vi "test appel.vi"() -> ()   [LabVIEW 2011]
uses:
  My DLL/Ap_int_usb.dll
panel:
  in  "Stop Button":bool
  out "Graphe":u16[](graph)
  out "Version DLL":i32
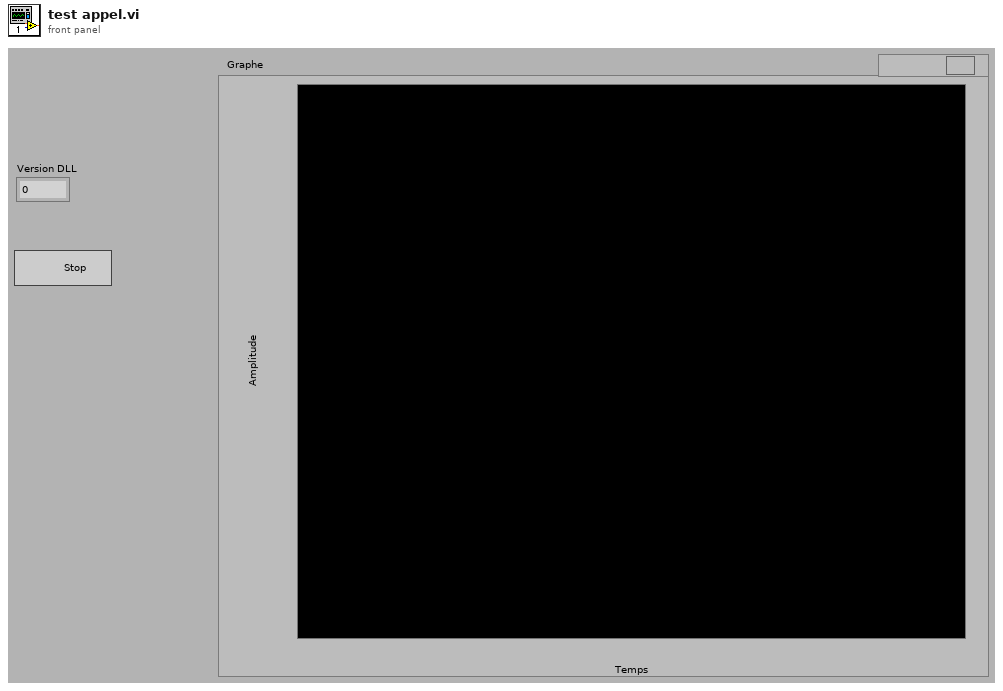
[diagram p1: front panel]
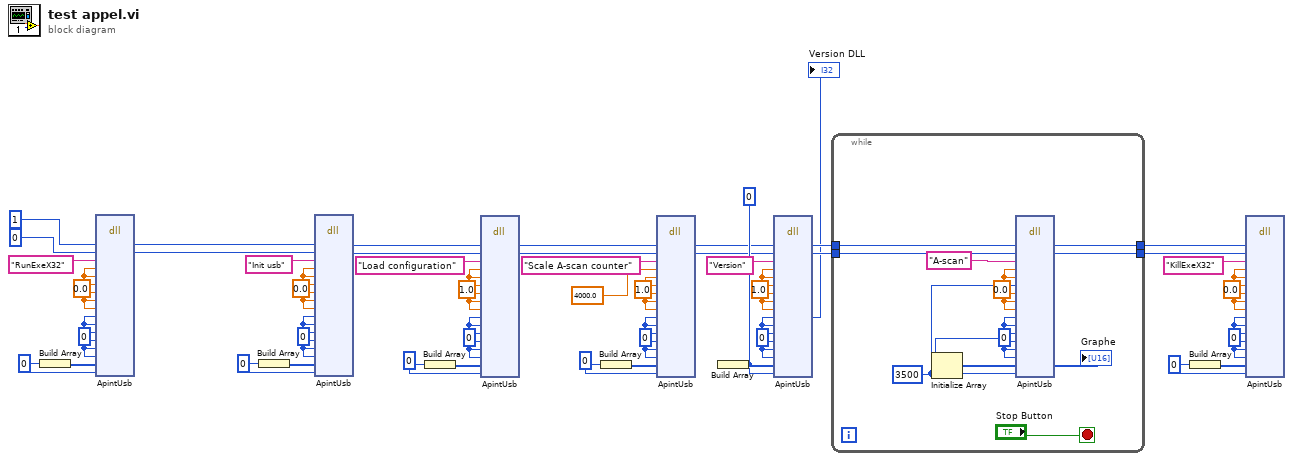
[diagram p0: block diagram]
diagram:
  w7 = u16 0 ("élément")
  w9 = i16 0 ("Out1")
  w10 = 1.0 ("In1")
  w14 = u16 0 ("élément")
  w16 = i16 0 ("Out1")
  w17 = 0.0 ("In1")
  w22 = u16 0 ("élément")
  w24 = i16 0 ("Out1")
  w25 = 0.0 ("In1")
  w30 = u16 0 ("élément")
  w32 = i16 0 ("Out1")
  w33 = 1.0 ("In1")
  w35 = u16 0 ("élément")
  w39 = i16 0 ("Out1")
  w40 = 1.0 ("In1")
  w42 = u16 0 ("élément")
  w44 = i16 0 ("Out1")
  w45 = 0.0 ("In1")
  n1 = Build Array(w22) -> (w23:u16[])
  n2 = dll-call lib="C:/Labview/Madelin/V2     LV2011 x64/DLL_Ap_int_usb   LV2011 x64/My DLL/Ap_int_usb.dll" fn="ApintUsb"("ProductNumber"=u32 1, "ChannelNumber"=u32 0, "Function"="RunExeX32", "In1"=w25, "In2"=w25, "In3"=w25, "In4"=w25, "In5"=w25, "In6"=w25, "Out1"=w24, "Out2"=w24, "Out3"=w24, "Out4"=w24, "Out5"=w24, "Out6"=w24, "Array"=w23, "Len"=w22) -> ("ProductNumber"=w19:u32, "ChannelNumber"=w1:u32)  [unwired: 19 in, 2 out]
  n3 = Build Array(w42) -> (w43:u16[])
  n4 = dll-call lib="C:/Labview/Madelin/V2     LV2011 x64/DLL_Ap_int_usb   LV2011 x64/My DLL/ap_int_usb.dll" fn="ApintUsb"("ProductNumber"=w19, "ChannelNumber"=w1, "Function"="Init usb", "In1"=w45, "In2"=w45, "In3"=w45, "In4"=w45, "In5"=w45, "In6"=w45, "Out1"=w44, "Out2"=w44, "Out3"=w44, "Out4"=w44, "Out5"=w44, "Out6"=w44, "Array"=w43, "Len"=w42) -> ("ProductNumber"=w37:u32, "ChannelNumber"=w36:u32)  [unwired: 19 in, 2 out]
  n5 = Build Array(w35) -> (w38:u16[])
  n6 = dll-call lib="C:/Labview/Madelin/V2     LV2011 x64/DLL_Ap_int_usb   LV2011 x64/My DLL/ap_int_usb.dll" fn="ApintUsb"("ProductNumber"=w37, "ChannelNumber"=w36, "Function"="Load configuration", "In1"=w40, "In2"=w40, "In3"=w40, "In4"=w40, "In5"=w40, "In6"=w40, "Out1"=w39, "Out2"=w39, "Out3"=w39, "Out4"=w39, "Out5"=w39, "Out6"=w39, "Array"=w38, "Len"=w35) -> ("ProductNumber"=w6:u32, "ChannelNumber"=w5:u32)  [unwired: 19 in, 2 out]
  n7 = Build Array(w7) -> (w8:u16[])
  n8 = dll-call lib="C:/Labview/Madelin/V2     LV2011 x64/DLL_Ap_int_usb   LV2011 x64/My DLL/Ap_int_usb.dll" fn="ApintUsb"("ProductNumber"=w6, "ChannelNumber"=w5, "Function"="Scale A-scan counter", "In1"=4000.0, "In2"=w10, "In3"=w10, "In4"=w10, "In5"=w10, "In6"=w10, "Out1"=w9, "Out2"=w9, "Out3"=w9, "Out4"=w9, "Out5"=w9, "Out6"=w9, "Array"=w8, "Len"=w7) -> ("ProductNumber"=w4:u32, "ChannelNumber"=w3:u32)  [unwired: 19 in, 2 out]
  n9 = Build Array(w30) -> (w31:u16[])
  n10 = dll-call lib="C:/Labview/Madelin/V2     LV2011 x64/DLL_Ap_int_usb   LV2011 x64/My DLL/ap_int_usb.dll" fn="ApintUsb"("ProductNumber"=w4, "ChannelNumber"=w3, "Function"="Version", "In1"=w33, "In2"=w33, "In3"=w33, "In4"=w33, "In5"=w33, "In6"=w33, "Out1"=w32, "Out2"=w32, "Out3"=w32, "Out4"=w32, "Out5"=w32, "Out6"=w32, "Array"=w31, "Len"=w30) -> ("ProductNumber"=w29:u32, "ChannelNumber"=w28:u32, "Out1"=→"Version DLL":i16)  [unwired: 18 in, 2 out]
  n11 = while {
    tunnel: w28 -> [w52]
    tunnel: w29 -> [w51]
    tunnel: [w49] -> w13
    tunnel: [w48] -> w12
    stop <- "Stop Button" stop-if-true
    w53 = 3500 ("taille de la dimension")
    w55 = i16 0 ("Out1")
    w56 = 0.0 ("In1")
    n12 = Initialize Array(w55, w53) -> (w54:i16[])
    n13 = dll-call lib="C:/Labview/Madelin/V2     LV2011 x64/DLL_Ap_int_usb   LV2011 x64/My DLL/ap_int_usb.dll" fn="ApintUsb"("ProductNumber"=w51, "ChannelNumber"=w52, "Function"="A-scan", "In1"=w56, "In2"=w56, "In3"=w53, "In4"=w56, "In5"=w56, "In6"=w56, "Out1"=w55, "Out2"=w55, "Out3"=w55, "Out4"=w55, "Out5"=w55, "Out6"=w55, "Array"=w54, "Len"=w53) -> ("ProductNumber"=w49:u32, "ChannelNumber"=w48:u32, "Array"=→"Graphe":u16[])  [unwired: 18 in, 2 out]
  }
  n14 = Build Array(w14) -> (w15:u16[])
  n15 = dll-call lib="C:/Labview/Madelin/V2     LV2011 x64/DLL_Ap_int_usb   LV2011 x64/My DLL/Ap_int_usb.dll" fn="ApintUsb"("ProductNumber"=w13, "ChannelNumber"=w12, "Function"="KillExeX32", "In1"=w17, "In2"=w17, "In3"=w17, "In4"=w17, "In5"=w17, "In6"=w17, "Out1"=w16, "Out2"=w16, "Out3"=w16, "Out4"=w16, "Out5"=w16, "Out6"=w16, "Array"=w15, "Len"=w14) -> ()  [unwired: 21 in, 2 out]
